vi "DMA.Scatter-Gather.Create Block Descriptors.vi"(8 "error in (no error)":errorcluster, 11 "GE 5565 params":T3 {"DMA Blocks"."size" format="%08x"; "DMA Blocks"."pointer" format="%08x"}) -> (0 "error out":errorcluster, 2 "block descriptors":T1[](array[typedef]) {"Block Descriptor"."next descriptor ptr" format="%08x"; "Block Descriptor"."data size" format="%08x"; "Block Descriptor"."data ptr (upper)" format="%08x"; "Block Descriptor"."data ptr (lower)" format="%08x"; "Block Descriptor"."descriptor ptr (aligned)" format="%08x"; "Block Descriptor"."descriptor size" format="%08x"; "Block Descriptor"."descriptor ptr (VISA)" format="%08x"; "VISA size" format="%08x"; "VISA offset" format="%08x"}, 3 "GE 5565 params out":T3 {"DMA Blocks"."size" format="%08x"; "DMA Blocks"."pointer" format="%08x"})   [LabVIEW 2016, in "GE 5565PIORC.lvclass"]
uses:
  GE 5565PIORC.lvclass
  Controls/GE 5565 Params.ctl
  Controls/DMA Block.ctl
  Controls/DMA Config.ctl
  Controls/DMA Block Descriptor (VISA).ctl
  Controls/DMA Block Descriptor.ctl
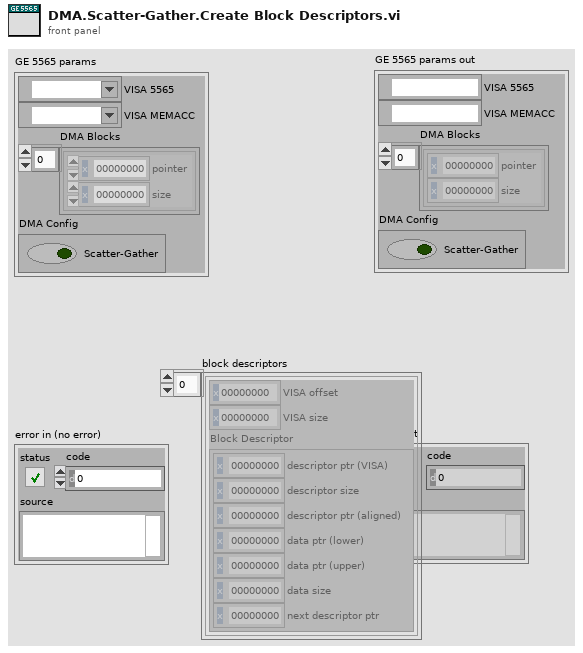
[diagram p1: front panel]
types:
  T1 = typedef "GE 5565PIORC.lvclass/DMA Block Descriptor (VISA).ctl" = cluster{"VISA offset":u32, "VISA size":u32, "Block Descriptor":T2}
  T2 = typedef "GE 5565PIORC.lvclass/DMA Block Descriptor.ctl" = cluster{"descriptor ptr (VISA)":u32, "descriptor size":u32, "descriptor ptr (aligned)":u32, "data ptr (lower)":u32, "data ptr (upper)":u32, "data size":u32, "next descriptor ptr":u32}
  T3 = typedef "GE 5565PIORC.lvclass/GE 5565 Params.ctl" = cluster{"VISA 5565":refnum<visa-resource-name>, "VISA MEMACC":refnum<visa-resource-name>, "DMA Blocks":T4[], "DMA Config":T5}
  T4 = typedef "GE 5565PIORC.lvclass/DMA Block.ctl" = cluster{"pointer":u32, "size":u32}
  T5 = typedef "GE 5565PIORC.lvclass/DMA Config.ctl" = cluster{"Scatter-Gather":bool}
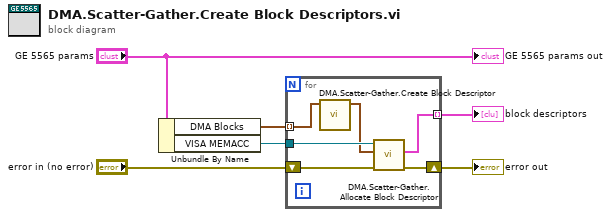
[diagram p0: block diagram]
diagram:
  n1 = Unbundle By Name("GE 5565 params") -> ("DMA Blocks"=w3:T4[], "VISA MEMACC"=w4:refnum<visa-resource-name>)
  n2 = for {
    shift-right: [w11] -> w5
    shift-left: "error in (no error)" -> [w12]
    tunnel: w3 -> [w9] mode=indexing
    tunnel: [w7] -> w2 mode=indexing
    tunnel: w4 -> [w10]
    n3 = call "DMA.Scatter-Gather.Create Block Descriptor.vi"("block"=w9) -> ("block descriptor"=w8:T2)  [unwired: 10 in]
    n4 = call "DMA.Scatter-Gather.Allocate Block Descriptor.vi"("error in (no error)"=w12, "block descriptor"=w8, "VISA Refnum in"=w10) -> ("error out"=w11:errorcluster, "allocated block descriptor"=w7:T1)  [unwired: 6 in, 1 out]
  }
  "error out" <- w5
  "block descriptors" <- w2
  "GE 5565 params out" <- "GE 5565 params"
